vi "Auto Drive Distance.vi"(0 "Wanted Distance":dbl, 1 "Left Gear Encoder":string, 2 "Right Gear Encoder":string, 3 "Reverse?":bool, 4 "1M in Distance":dbl) -> (5 "Left Stick Value":dbl, 6 "Right Stick Value":dbl, 7 "Completed?":bool)   [LabVIEW 2012]
panel:
  # "Tank Drive ONLY"
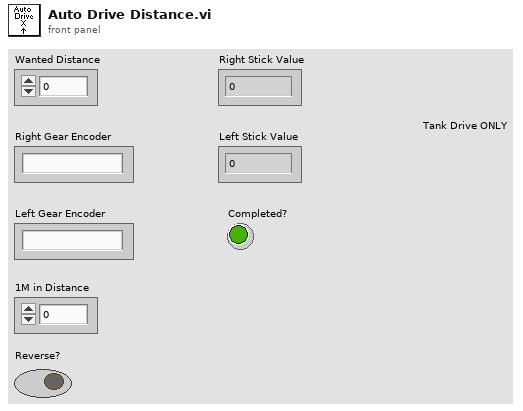
[diagram p1: front panel]
types:
  T1 = typedef "WPI_EncoderDevRef.ctl" = cluster{"DevStatus":errorcluster, "EncoderIndex":T2, "CounterIndex":T3, "DistancePerCount":dbl, "Decoding Type":T4}
  T2 = typedef "FPGA_EncoderIdx.ctl" = enum8{"Enc 0", "Enc 1", "Enc 2", "Enc 3", "Invalid"}
  T3 = typedef "FPGA_CounterCtrSystemIndex.ctl" = enum8{"Ctr 0", "Ctr 1", "Ctr 2", "Ctr 3", "Ctr 4", "Ctr 5", "Ctr 6", "Ctr 7", "Invalid"}
  T4 = typedef "WPI_EncoderType.ctl" = enum16{"1x", "2x", "4x"}
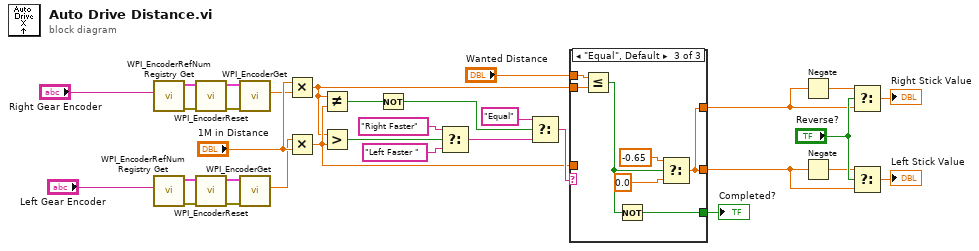
[diagram p0: block diagram]
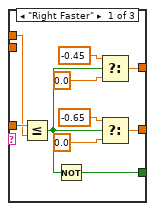
[diagram p2: hidden frame]
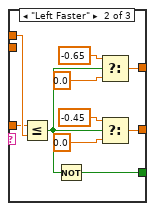
[diagram p3: hidden frame]
diagram:
  n1 = call <vilib>:"WPI_EncoderRefNum Registry Get.vi"("refnum name"="Right Gear Encoder") -> ("error out"=w14:errorcluster, "EncoderDevRef"=w15:T1)  [unwired: 9 in]
  n2 = call <vilib>:"WPI_EncoderRefNum Registry Get.vi"("refnum name"="Left Gear Encoder") -> ("error out"=w9:errorcluster, "EncoderDevRef"=w10:T1)  [unwired: 9 in]
  n3 = call <vilib>:"WPI_EncoderReset.vi"("error in (no error)"=w14, "EncoderDevRef"=w15) -> ("error out"=w12:errorcluster, "EncoderDevRef"=w13:T1)  [unwired: 8 in]
  n4 = call <vilib>:"WPI_EncoderReset.vi"("error in (no error)"=w9, "EncoderDevRef"=w10) -> ("error out"=w8:errorcluster, "EncoderDevRef"=w11:T1)  [unwired: 8 in]
  n5 = call <vilib>:"WPI_EncoderGet.vi"("error in (no error)"=w12, "EncoderDevRef"=w13) -> ("Distance"=w17:dbl)  [unwired: 4 in, 5 out]
  n6 = call <vilib>:"WPI_EncoderGet.vi"("error in (no error)"=w8, "EncoderDevRef"=w11) -> ("Distance"=w19:dbl)  [unwired: 4 in, 5 out]
  n7 = Multiply(x="1M in Distance", y=w17) -> (x*y=w16:dbl)
  n8 = Multiply(x=w19, y="1M in Distance") -> (x*y=w18:dbl)
  n9 = Not Equal?(x=w16, y=w18) -> (x != y?=w29:bool)
  n10 = Greater?(x=w16, y=w18) -> (0:w27:bool)
  n11 = Not(x=w29) -> (.not. x?=w30:bool)
  n12 = Select(t="Right Faster", s=w27, f="Left Faster ") -> (s? t:f=w24:string)
  n13 = Select(t="Equal", s=w30, f=w24) -> (s? t:f=w23:string)
  n14 = case shown="\"Equal\", Default" w23 {
    tunnel: "Wanted Distance" -> [w39 w48 w54]
    tunnel: w16 -> [_ _ w59]
    tunnel: [w37 w50 w56] -> w21
    tunnel: [w34 w44 w53] -> w3
    tunnel: [w38 w49 w53] -> w5
    tunnel: w18 -> [w40 w47 _]
    frame "Right Faster" {
      n15 = Less Or Equal?(x=w40, y=w39) -> (x <= y?=w35:bool)
      n16 = Not(x=w35) -> (.not. x?=w37:bool)
      n17 = Select(t=-0.45, s=w35, f=0.0) -> (s? t:f=w34:dbl)
      n18 = Select(t=-0.65, s=w35, f=0.0) -> (s? t:f=w38:dbl)
    }
    frame "Left Faster" {
      n19 = Less Or Equal?(x=w47, y=w48) -> (x <= y?=w43:bool)
      n20 = Not(x=w43) -> (.not. x?=w50:bool)
      n21 = Select(t=-0.65, s=w43, f=0.0) -> (s? t:f=w44:dbl)
      n22 = Select(t=-0.45, s=w43, f=0.0) -> (s? t:f=w49:dbl)
    }
    frame "Equal", Default {
      n23 = Less Or Equal?(x=w54, y=w59) -> (x <= y?=w57:bool)
      n24 = Not(x=w57) -> (.not. x?=w56:bool)
      n25 = Select(t=-0.65, s=w57, f=0.0) -> (s? t:f=w53:dbl)
    }
  }
  "Completed?" <- w21
  n26 = Negate(x=w3) -> (-x=w4:dbl)
  n27 = Negate(x=w5) -> (-x=w6:dbl)
  n28 = Select(t=w4, s="Reverse?", f=w3) -> (s? t:f=→"Right Stick Value":dbl)
  n29 = Select(t=w6, s="Reverse?", f=w5) -> (s? t:f=→"Left Stick Value":dbl)
